vi "CSTK_MCListbox Designer.vi"   [LabVIEW 2015]
uses:
  Library/MCListbox Designer/CSTK_MCListbox_Designer.vi
  Library/MCListbox Designer/CSTK_MCListbox Designer.lvlib
panel:
  # "MCListbox Designer"
types:
  T1 = enum32{"Invalid", "Standard", "Closed", "Hidden", "Minimized", "Maximized"}
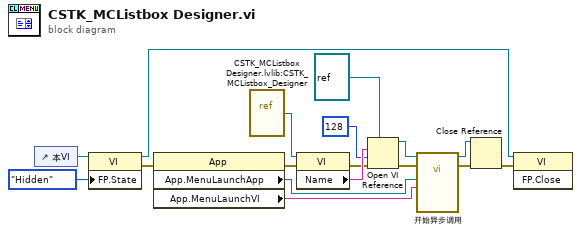
[diagram p0: block diagram]
diagram:
  n1 = control-ref of="本VI"() -> (w16:refnum<vi>)
  n2 = property class="VI"(reference=w16, "FP.State"=T1."Hidden" ("前面板窗口:状态")) -> (reference out=w2:refnum<vi>, error out=w5:errorcluster)  [unwired: 1 in]
  n3 = property class="App"(error in=w5) -> (error out=w4:errorcluster, "App.MenuLaunchApp"=w7:refnum<vi>, "App.MenuLaunchVI"=w6:string)  [unwired: 1 in, 1 out]
  n4 = vi-ref "CSTK_MCListbox Designer.lvlib:CSTK_MCListbox_Designer.vi"() -> (w14:refnum<vi>)
  n5 = property class="VI"(reference=w14, error in=w4) -> (error out=w8:errorcluster, "Name"=w17:string)  [unwired: 1 out]
  n6 = Open VI Reference(type specifier VI Refnum (for type only)=refnum<vi> refnum ("类型说明符VI引用句柄（仅用于类型）"), vi path=w17, options=128 ("选项"), error in (no error)=w8) -> (vi reference=w12:refnum<vi>, error out=w11:errorcluster)  [unwired: 2 in]
  n7 = call-by-ref "开始异步调用"(reference=w12, error in=w11, "应用程序:菜单启动:VI"=w6, "应用程序引用（本地）"=w7) -> (reference out=w10:refnum<vi>, error out=w9:errorcluster)  [unwired: 10 in]
  n8 = Close Reference(reference=w10, error in (no error)=w9) -> (error out=w1:errorcluster)
  n9 = invoke class="VI" method="FP.Close"(reference=w2, error in=w1) -> ()  [unwired: 1 in, 3 out]
